vi "Open.vi"(0 "2-channel USB 3.0 device on non-USB 3.0 Port":bool, 7 "Serial Number":string, 8 "4-channel USB Powered":bool, 9 "Resolution":i32(ring) items=["8-bit", "12-bit", "14-bit", "15-bit (max. 2 ch.)", "16-bit (max. 1 ch.)"], 10 "Use Serial Number":bool) -> (1 "USB Powered Indication":bool, 2 "handle":i16, 4 "Max ADC value":i16, 5 "2-channel USB 3.0 device on non-USB 3.0 Port Indication":bool, 6 "Device Info":T1)   [LabVIEW 2017]
doc: "This VI opens a PicoScope 3000a/b and returns a handle to the device."
uses:
  ps5000a.dll
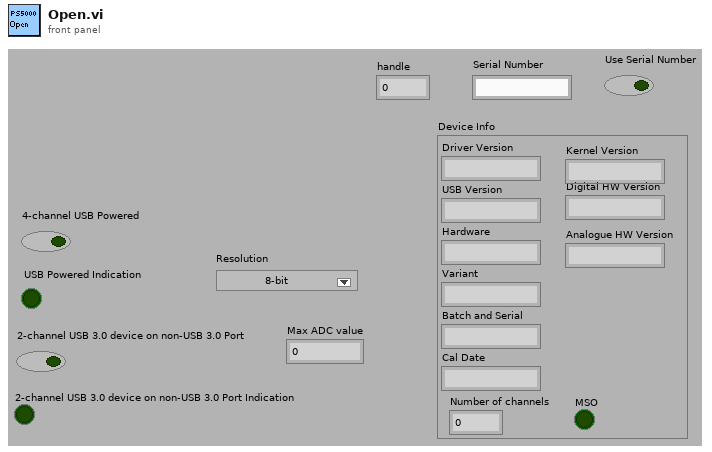
[diagram p1: front panel]
types:
  T1 = cluster{"Driver Version":string, "USB Version":string, "Hardware":string, "Variant":string, "Batch and Serial":string, "Cal Date":string, "Kernel Version":string, "Digital HW Version":string, "Analogue HW Version":string, "MSO":bool, "Number of channels":i16}
  T2 = cluster{"Driver Version":string, "USB Version":string, "Hardware":string, "Variant":string, "Batch and Serial":string, "Cal Date":string, "Kernel Version":string, "Digital HW Version":string, "Analogue HW Version":string, "Firmware 1":string, "Firmware 2":string}
  T3 = cluster{"Driver Version":string, "USB Version":string, "Hardware":string, "Variant":string, "Batch and Serial":string, "Cal Date":string, "Kernel Version":string, "Digital HW Version":string, "Analogue HW Version":string, bool, i16}
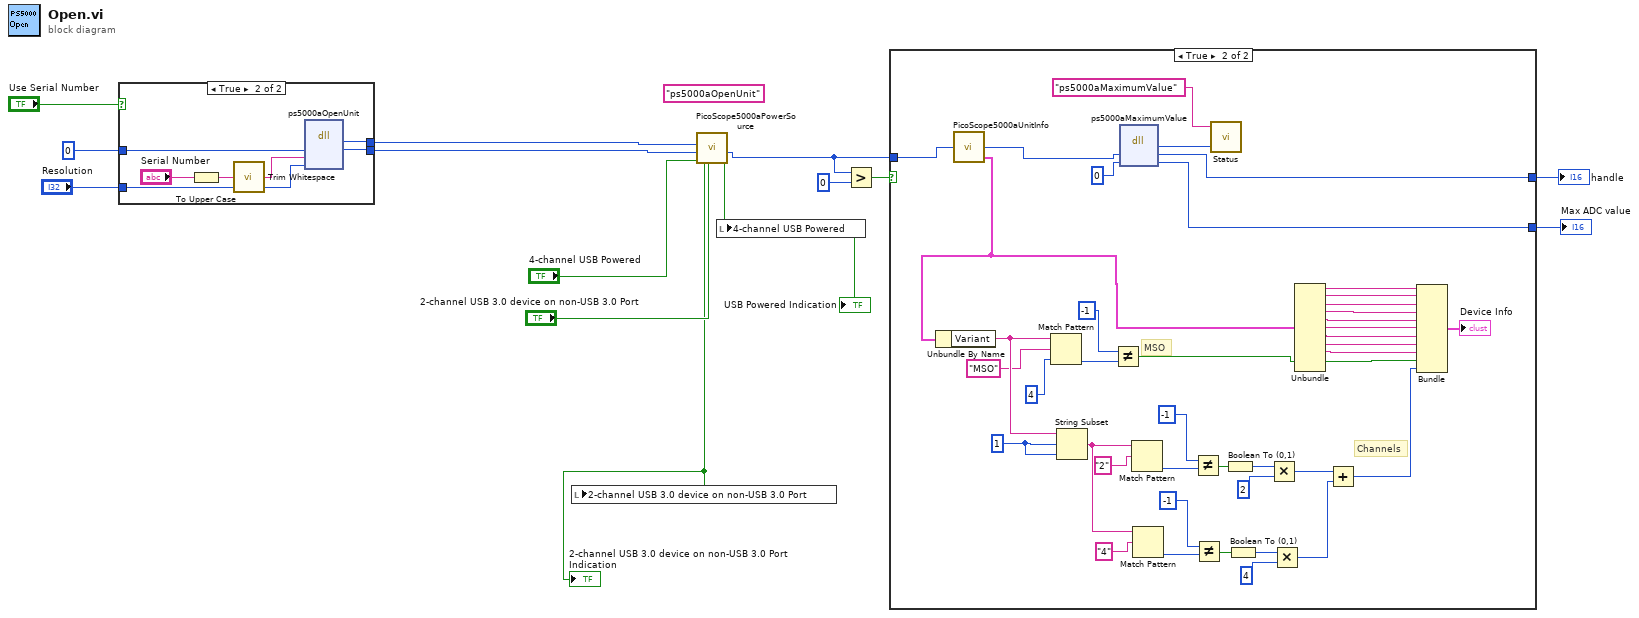
[diagram p0: block diagram]
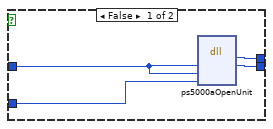
[diagram p2: hidden frame]
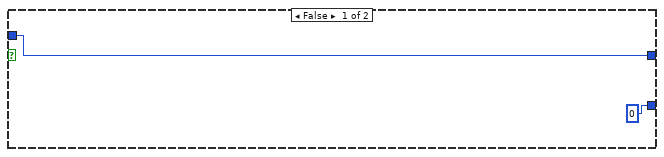
[diagram p3: hidden frame]
diagram:
  (unwired) "ps5000aOpenUnit" ("source")
  n1 = case shown="True" "Use Serial Number" {
    tunnel: i16 0 ("handle") -> [w15 w23]
    tunnel: [w18 w25] -> w13
    tunnel: [w17 w24] -> w12
    tunnel: "Resolution" -> [w16 w22]
    frame False {
      n2 = dll-call lib="ps5000a.dll" fn="ps5000aOpenUnit" ("ps3000.dll:_ps3000_open_unit@0")("handle"=w15, "serial"=w15, "resolution"=w16) -> ("PICO_STATUS"=w18:i32, "handle"=w17:i16)  [unwired: 5 in, 2 out]
    }
    frame True {
      n3 = To Upper Case(1:"Serial Number") -> (0:w20:string)
      n4 = call <vilib>:"Trim Whitespace.vi"("string"=w20) -> ("trimmed string"=w19:string)  [unwired: 1 in]
      n5 = dll-call lib="ps5000a.dll" fn="ps5000aOpenUnit" ("ps3000.dll:_ps3000_open_unit@0")("handle"=w23, "serial"=w19, "resolution"=w22) -> ("PICO_STATUS"=w25:u32, "handle"=w24:i16)  [unwired: 5 in, 2 out]
    }
  }
  n6 = call "PicoScope5000aPowerSource.vi"("USB 3.0 on non-USB 3.0 port"="2-channel USB 3.0 device on non-USB 3.0 Port", "USB Powered"="4-channel USB Powered", "handle in"=w12, "PICO STATUS IN"=w13) -> ("USB Powered Indicator"=w10:bool, "handle out"=w7:i16, "USB 3 Indicator"=w1:bool)  [unwired: 3 in, 2 out]
  "USB Powered Indication" <- w10
  "2-channel USB 3.0 device on non-USB 3.0 Port Indication" <- w1
  n7 = local write "2-channel USB 3.0 device on non-USB 3.0 Port"(w1) -> ()
  n8 = local write "4-channel USB Powered"(w10) -> ()
  n9 = Greater?(x=w7, y=0) -> (0:w8:bool)
  n10 = case shown="True" w8 {
    tunnel: w7 -> [w27 w68]
    tunnel: [w27 w31] -> w9
    tunnel: [i16 0 ("value") w29] -> w3
    frame False {
    }
    frame True {
      w58 = 1 ("offset (0)")
      # "MSO"
      # "Channels"
      n11 = call "PicoScope5000aUnitInfo.vi"("handle in"=w68) -> ("Unit Info"=w34:T2, "handle out"=w33:i16)  [unwired: 2 in, 1 out]
      n12 = Unbundle By Name(w34) -> ("Variant"=w54:string)
      n13 = Match Pattern(string=w54, regular expression="MSO", offset (0)=4) -> (offset past match=w51:i32)  [unwired: 3 out]
      n14 = String Subset(string=w54, offset (0)=w58, length (rest)=w58) -> (substring=w45:string)
      n15 = Not Equal?(x=-1, y=w51) -> (x != y?=w49:bool)
      n16 = dll-call lib="ps5000a.dll" fn="ps5000aMaximumValue"("handle"=w33, "value"=i16 0) -> ("PICO_STATUS"=w32:u32, "handle"=w31:i16, "value"=w29:i16)  [unwired: 3 in, 2 out]
      n17 = Match Pattern(string=w45, regular expression="2") -> (offset past match=w56:i32)  [unwired: 1 in, 3 out]
      n18 = Match Pattern(string=w45, regular expression="4") -> (offset past match=w47:i32)  [unwired: 1 in, 3 out]
      n19 = Not Equal?(x=-1, y=w56) -> (x != y?=w41:bool)
      n20 = Not Equal?(x=-1, y=w47) -> (x != y?=w37:bool)
      n21 = call "Status.vi"("PICO STATUS"=w32, "source"="ps5000aMaximumValue") -> ()  [unwired: 1 in, 1 out]
      n22 = Boolean To (0,1)(Boolean=w41) -> (0, 1=w40:i16)
      n23 = Boolean To (0,1)(Boolean=w37) -> (0, 1=w38:i16)
      n24 = Multiply(x=w40, y=i16 2) -> (x*y=w44:i16)
      n25 = Multiply(x=w38, y=i16 4) -> (x*y=w36:i16)
      n26 = Unbundle(w34) -> ("Driver Version"=w67:string, "USB Version"=w66:string, "Hardware"=w65:string, "Variant"=w64:string, "Batch and Serial"=w63:string, "Cal Date"=w62:string, "Kernel Version"=w61:string, "Digital HW Version"=w60:string, "Analogue HW Version"=w59:string)  [unwired: 2 out]
      n27 = Add(x=w44, y=w36) -> (x+y=w43:i16)
      n28 = Bundle("Driver Version"=w67, "USB Version"=w66, "Hardware"=w65, "Variant"=w64, "Batch and Serial"=w63, "Cal Date"=w62, "Kernel Version"=w61, "Digital HW Version"=w60, "Analogue HW Version"=w59, w49, w43) -> (→"Device Info":T3)  [unwired: 1 in]
    }
  }
  "handle" <- w9
  "Max ADC value" <- w3
